vi "LoadDataHH.vi"(5 "Path":refnum<vi>) -> (0 "gap photons":u32, 1 "invalid photons":u32, 2 "total":u32)   [LabVIEW 2009]
panel:
  out "% done":dbl(slide) scale=0.0..100.0
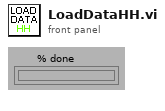
[diagram p1: front panel]
types:
  T1 = typedef "FIFOSettings_BH.ctt" = cluster{"Measurement":cluster{"Binning (ms)":sgl, "External Trigger Condition":u16, "Stop Condition:":u16, "Stop Count":dbl, "Buffer Size (Photons)":u16, "No of Channels":u16, "Ext Latch Delay":i16}, "ADC":cluster{"Module":u16, "ADC Resolution":i32, "Dither Range":i16, "Count Increment":i16, "Macro Time Clock":i16}, "SYNC":cluster{"SYNC ZC Level (mV)":sgl, "SYNC Freq Divider":i16, "SYNC Holdoff (ns)":sgl, "SYNC Threshold (mV)":sgl}, "TAC":cluster{"TAC Range (ns)":sgl, "TAC Gain":i16, "TAC Offset (%)":sgl, "TAC Limit Low (%)":sgl, "TAC Limit High (%)":sgl}, "CFD":cluster{"CFD Limit Low (mV)":sgl, "CFD Limit High (mV)":sgl, "CFD ZC Level (mV)":sgl, "CFD Holdoff (ns)":sgl}}
  T2 = cluster{"router channels":u8[], "macro times(50ns steps)":u32[], "micro times":u16[], "invalid times":u32[], "gap times":u32[]}
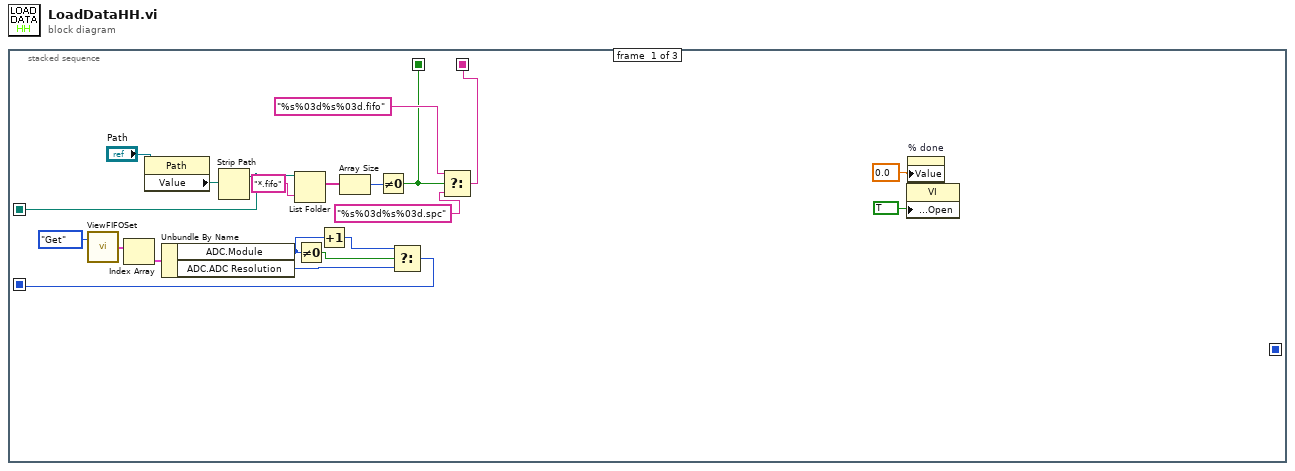
[diagram p0: block diagram]
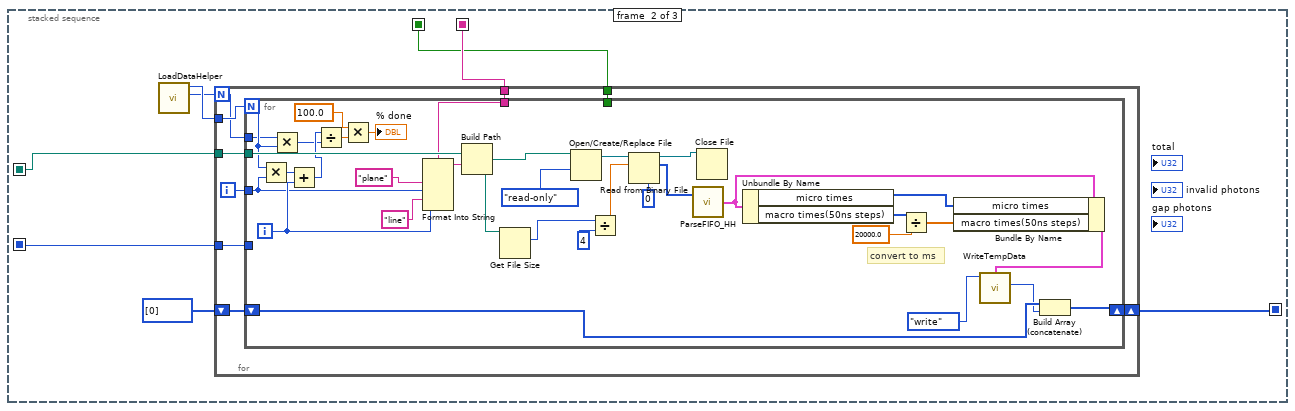
[diagram p2: hidden frame]
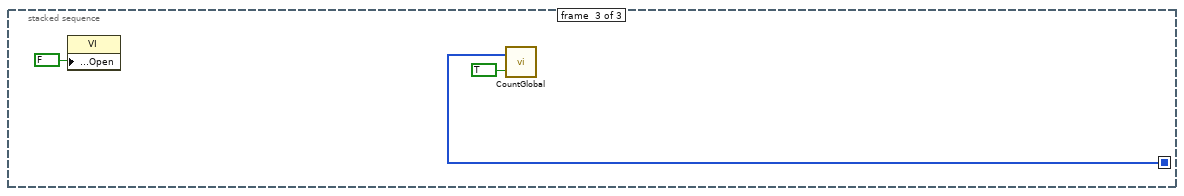
[diagram p3: hidden frame]
diagram:
  n1 = stacked-sequence {
    seq-local: [_ w27 _] -> [_ _ w74]
    seq-local: [w12 _ _] -> [_ w24 _]
    seq-local: [w2 _ _] -> [_ w23 _]
    seq-local: [w8 _ _] -> [_ w22 _]
    seq-local: [w1 _ _] -> [_ w21 _]
    frame #0 {
      n2 = call "ViewFIFOSet.vi"("Enum"=enum16{"Display", "change", "Get", "Set"}."Get") -> ("FIFO Settings (Array)"=w17:T1[])  [unwired: 1 in]
      n3 = Index Array(array=w17) -> (element=w16:T1)  [unwired: 1 in]
      n4 = property on="Property Node" class="Path"(reference="Path") -> ("Value"=w10:path)  [unwired: 1 in, 2 out]
      n5 = Unbundle By Name(w16) -> ("ADC.Module"=w13:u16, "ADC.ADC Resolution"=w15:i32)
      n6 = Strip Path(path=w10) -> (stripped path=w8:path)  [unwired: 1 out]
      n7 = List Folder(path=w8, pattern="*.fifo") -> (filenames=w6:string[])  [unwired: 2 in, 3 out]
      n8 = Not Equal To 0?(x=w13) -> (x != 0?=w14:bool)
      n9 = Increment(x=w13) -> (x+1=w11:u16)
      n10 = Array Size(array=w6) -> (size(s)=w5:i32)
      n11 = Not Equal To 0?(x=w5) -> (x != 0?=w1:bool)
      n12 = Select(t=w11, s=w14, f=w15) -> (s? t:f=w12:i32)
      n13 = Select(t="%s%03d%s%03d.fifo" ("format string"), s=w1, f="%s%03d%s%03d.spc" ("format string")) -> (s? t:f=w2:string)
      n14 = property class="VI"("Front Panel Window:Open"=TRUE) -> ()  [unwired: 2 in, 2 out]
      n15 = property on="% done" class="Slide (strict)"("Value"=0.0 ("% done")) -> ()  [unwired: 2 in, 2 out]
    }
    frame #1 {
      n16 = call "LoadDataHelper.vi"() -> ("planes"=w25:u32, "lines"=w26:u32)  [unwired: 7 in, 3 out]
      n17 = for {
        N: w25 -> [w31]
        tunnel: w26 -> [w34]
        tunnel: w22 -> [w37]
        tunnel: w24 -> [w35]
        shift-right: [w32] -> w27
        shift-left: i32[] [0] -> [w33]
        tunnel: w23 -> [w30]
        tunnel: w21 -> [w29]
        i -> [w36]
        n18 = for {
          N: w34 -> [w58]
          tunnel: w37 -> [w71]
          tunnel: w36 -> [w61]
          tunnel: w35 -> [_]
          shift-right: [w69] -> w32
          shift-left: w33 -> [w70]
          tunnel: w31 -> [w57]
          tunnel: w30 -> [w55]
          tunnel: w29 -> [_]
          i -> [w62]
          # "convert to ms"
          n19 = Multiply(x=w58, y=w61) -> (x*y=w59:i32)
          n20 = Multiply(x=w57, y=w58) -> (x*y=w56:i32)
          n21 = Add(x=w59, y=w62) -> (x+y=w60:i32)
          n22 = Divide(x=w60, y=w56) -> (x/y=w68:dbl)
          n23 = Multiply(x=100.0, y=w68) -> (x*y=→"% done":dbl)
          n24 = Format Into String(format string=w55, "plane", w61, "line", w62) -> (resulting string=w63:string)  [unwired: 2 in, 1 out]
          n25 = Build Path(base path=w71, name or relative path=w63) -> (appended path=w48:path)
          n26 = Get File Size(file=w48) -> (size (in bytes)=w45:i64)  [unwired: 1 in, 2 out]
          n27 = Open/Create/Replace File(file path (use dialog)=w48, access (0:read/write)=enum16{"read/write", "read-only", "write-only"}."read-only") -> (refnum out=w46:refnum<file>)  [unwired: 4 in, 2 out]
          n28 = Divide(x=w45, y=u8 4) -> (x/y=w51:dbl)
          n29 = Read from Binary File(5:u32 0 ("Byte-Stream-Typ"), 10:w51, 11:w46) -> (2:w52:u32[], 3:w44:refnum<file>)  [unwired: 3 in, 2 out]
          n30 = call "ParseFIFO_HH.vi"("RawData"=w52) -> ("RawData Out"=w41:T2)  [unwired: 1 in]
          n31 = Close File(refnum=w44) -> ()  [unwired: 1 in, 2 out]
          n32 = Unbundle By Name(w41) -> ("micro times"=w38:u16[], "macro times(50ns steps)"=w42:u32[])
          n33 = Divide(x=w42, y=20000.0) -> (x/y=w40:dbl[])
          n34 = Bundle By Name(cluster=w41, "micro times"=w38, "macro times(50ns steps)"=w40) -> (w39:T2)
          n35 = call "WriteTempData.vi"("rawdata"=w39, "Enum"=enum16{"create new", "write", "close"}."write") -> ("offset"=w53:i32)  [unwired: 3 in, 1 out]
          n36 = Build Array (concatenate)(w70, w53) -> (w69:i32[])
        }
      }
    }
    frame #2 {
      n37 = property class="VI"("Front Panel Window:Open"=FALSE) -> ()  [unwired: 2 in, 2 out]
      n38 = call "CountGlobal.vi"("changed?"=TRUE, "count"=w74) -> ()  [unwired: 1 in, 1 out]
    }
  }
